vi "Check Step Result.vi"(7 "Execution in":refnum<data-value>, 8 "error in (no error)":errorcluster, 9 "Skipped":bool, 10 "Output Values in":cluster{"Name":string, "Variant Data":variant}[](array[cluster]), 11 "Step in":refnum<class "Step.lvclass">) -> (0 "Error Info":string, 1 "Result":T5, 2 "Measure Results":T2[](array[typedef]), 3 "Step out":refnum<class "Step.lvclass">, 4 "Value Limit Data":T1, 5 "Execution out":refnum<data-value>)   [LabVIEW 2015, in "Execution.lvclass"]
uses:
  Execution.lvclass
  Step.lvclass
  Step/STEP_STATUS.ctl
  STEP_MEASURE_RESULT.ctl
  Step/OUTPUT_DATA_TYPE.ctl
  OutputUI/OUTPUT_CHECK_TYPE.ctl
  <vilib>/Utility/error.llb/DialogType.ctl
panel:
  out "Output Values out":cluster{"Name":string, "Variant Data":variant}[](array[cluster])
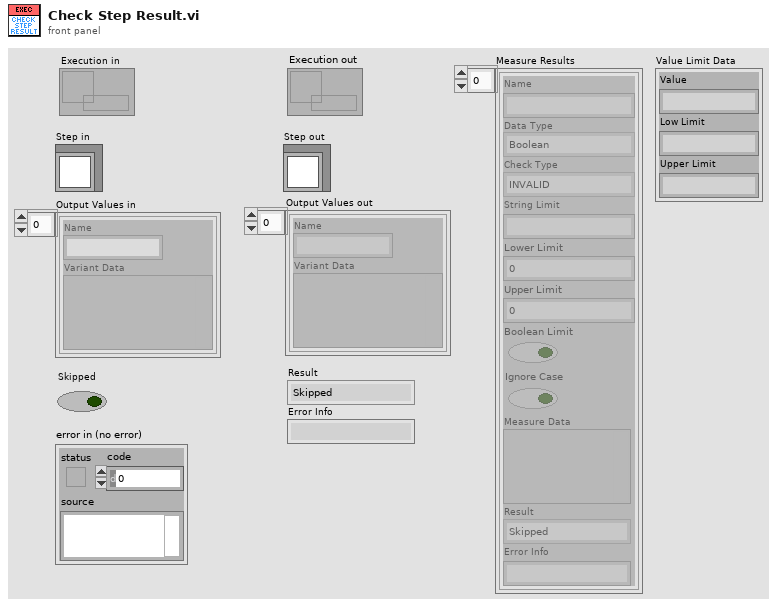
[diagram p1: front panel]
types:
  T1 = cluster{"Value":string, "Low Limit":string, "Upper Limit":string}
  T2 = typedef "Execution.lvclass/STEP_MEASURE_RESULT.ctl" = cluster{"Name":string, "Data Type":T3, "Check Type":T4, "String Limit":string, "Lower Limit":dbl, "Upper Limit":dbl, "Boolean Limit":bool, "Ignore Case":bool, "Measure Data":variant, "Result":T5, "Error Info":string}
  T3 = typedef "Step.lvclass/OUTPUT_DATA_TYPE.ctl" = enum16{"Boolean", "String", "Numeric", "Other"}
  T4 = typedef "Step.lvclass/OUTPUT_CHECK_TYPE.ctl" = enum16{"INVALID", "DO_NOT_CHECK", "RECORD", "VARIABLE", "EQUAL", "NOT_EQUAL", "STR_CONTAINS", "STR_START_WITH", "STR_END_WITH", "STR_REGEX_MATCH", "NUM_GT", "NUM_LT", "NUM_GE", "NUM_LE", "NUM_RANGE", "NUM_RANGE_BDY"}
  T5 = typedef "Step.lvclass/STEP_STATUS.ctl" = enum16{"Skipped", "Done", "Passed", "Failed", "Error"}
  T6 = typedef "Step.lvclass/STEP_OUTPUT.ctl" = cluster{"Label":string, "Name":string, "Data Type":T3, "Check Type":T4, "String Limit":string, "Lower Limit":dbl, "Upper Limit":dbl, "Boolean Limit":bool, "Ignore Case":bool, "Variable Name 1":string, "Limit Value Type 1":T7, "Variable Name 2":string, "Limit Value Type 2":T7}
  T7 = typedef "Step.lvclass/OUTPUT_VALUE_TYPE.ctl" = enum16{"Constant", "Variable"}
  T8 = typedef "DialogType.ctl" = u16
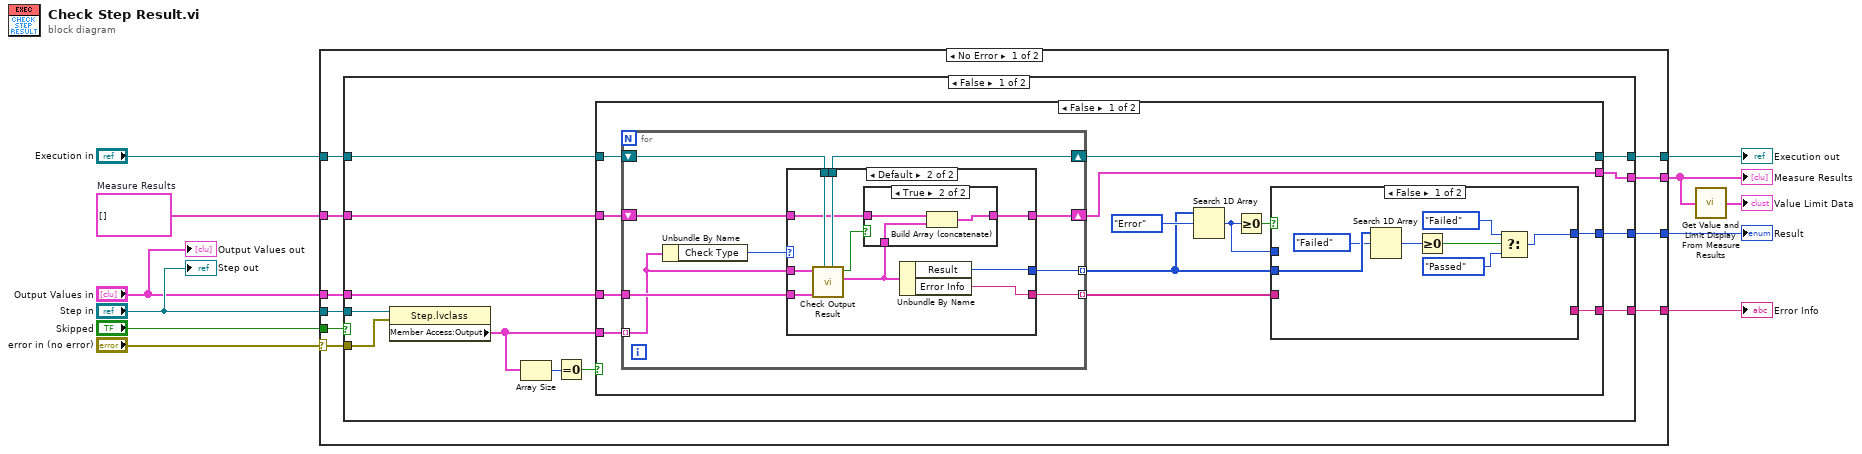
[diagram p0: block diagram]
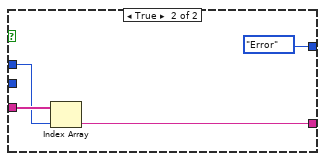
[diagram p2: hidden frame]
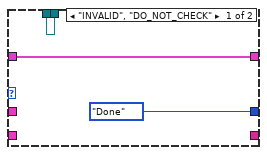
[diagram p3: hidden frame]
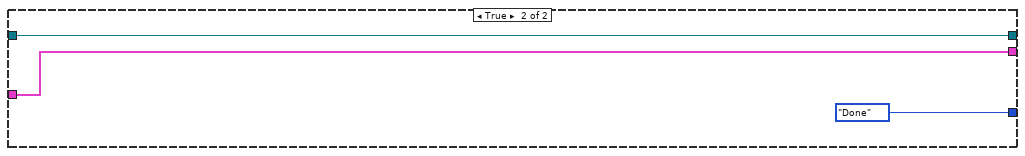
[diagram p5: hidden frame]
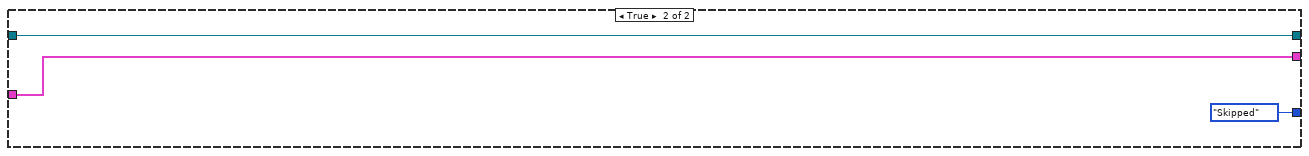
[diagram p6: hidden frame]
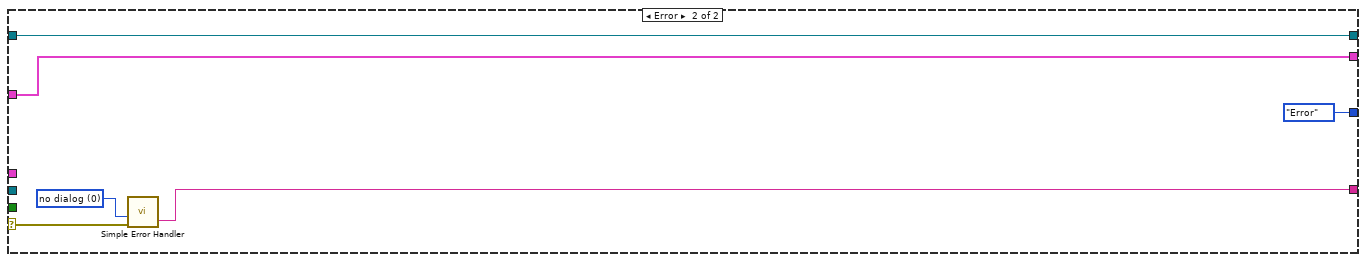
[diagram p7: hidden frame]
diagram:
  w3 = T2[] []  # Measure Results
  n1 = case shown="No Error" "error in (no error)" {
    selector: "error in (no error)" -> [w18 w94]
    tunnel: [w20 STEP_STATUS."Error" ("Status")] -> w10
    tunnel: [w16 w93] -> w9
    tunnel: "Skipped" -> [w21 _]
    tunnel: "Step in" -> [w19 _]
    tunnel: "Output Values in" -> [w17 _]
    tunnel: "Execution in" -> [w15 w91]
    tunnel: [w14 w91] -> w4
    tunnel: w3 -> [w13 w90]
    tunnel: [w12 w90] -> w2
    frame No Error {
      n2 = case shown="False" w21 {
        tunnel: [w29 STEP_STATUS."Skipped" ("Status")] -> w20
        tunnel: w19 -> [w33 _]
        tunnel: w18 -> [w32 _]
        tunnel: w17 -> [w27 _]
        tunnel: [w26 _] -> w16
        tunnel: w15 -> [w25 w88]
        tunnel: [w24 w88] -> w14
        tunnel: w13 -> [w23 w87]
        tunnel: [w22 w87] -> w12
        frame False {
          n3 = property class="Step.lvclass"(reference=w33, error in=w32) -> ("Member Access:Output"=w28:T6[])  [unwired: 2 out]
          n4 = Array Size(array=w28) -> (size(s)=w31:i32)
          n5 = Equal To 0?(x=w31) -> (x = 0?=w30:bool)
          n6 = case shown="False" w30 {
            tunnel: [w39 STEP_STATUS."Done" ("Status")] -> w29
            tunnel: w28 -> [w46 _]
            tunnel: w27 -> [w45 _]
            tunnel: [w38 _] -> w26
            tunnel: w25 -> [w37 w85]
            tunnel: [w36 w85] -> w24
            tunnel: w23 -> [w35 w84]
            tunnel: [w34 w84] -> w22
            frame False {
              n7 = for {
                tunnel: w46 -> [w61] mode=indexing
                tunnel: w45 -> [w66]
                tunnel: [w65] -> w40 mode=indexing
                tunnel: [w64] -> w41 mode=indexing
                shift-right: [w62] -> w36
                shift-left: w37 -> [w63]
                shift-right: [w58] -> w34
                shift-left: w35 -> [w59]
                n8 = Unbundle By Name(w61) -> ("Check Type"=w60:T4)
                n9 = case shown="Default" w60 {
                  tunnel: w61 -> [_ w79]
                  tunnel: w66 -> [_ w78]
                  tunnel: [STEP_STATUS."Done" ("Status") w72] -> w65
                  tunnel: [_ w71] -> w64
                  tunnel: w63 -> [w69 w77]
                  tunnel: [w69 w76] -> w62
                  tunnel: w59 -> [w67 w75]
                  tunnel: [w67 w74] -> w58
                  frame "INVALID", "DO_NOT_CHECK" {
                  }
                  frame Default {
                    n10 = call "Check Output Result.vi"("Execution in"=w77, "Output Values"=w78, "Step Output"=w79) -> ("Measure Result"=w73:T2, "Include In Result"=w70:bool, "Execution out"=w76:refnum<data-value>)  [unwired: 6 in]
                    n11 = case shown="True" w70 {
                      tunnel: w75 -> [w80 w83]
                      tunnel: [w80 w82] -> w74
                      tunnel: w73 -> [_ w81]
                      frame False {
                      }
                      frame True {
                        n12 = Build Array (concatenate)(w83, w81) -> (w82:T2[])
                      }
                    }
                    n13 = Unbundle By Name(w73) -> ("Result"=w72:T5, "Error Info"=w71:string)
                  }
                }
              }
              n14 = Search 1D Array(1D array=w40, element=STEP_STATUS."Error" ("Status")) -> (index of element=w42:i32)  [unwired: 1 in]
              n15 = Greater Or Equal To 0?(x=w42) -> (x >= 0?=w43:bool)
              n16 = case shown="False" w43 {
                tunnel: w42 -> [_ w56]
                tunnel: w41 -> [_ w57]
                tunnel: [w47 STEP_STATUS."Error" ("Status")] -> w39
                tunnel: [_ w54] -> w38
                tunnel: w40 -> [w53 _]
                frame False {
                  n17 = Search 1D Array(1D array=w53, element=STEP_STATUS."Failed" ("Status")) -> (index of element=w51:i32)  [unwired: 1 in]
                  n18 = Greater Or Equal To 0?(x=w51) -> (x >= 0?=w50:bool)
                  n19 = Select(t=STEP_STATUS."Failed" ("Status"), s=w50, f=STEP_STATUS."Passed" ("Status")) -> (s? t:f=w47:T5)
                }
                frame True {
                  n20 = Index Array(array=w57, index=w56) -> (element=w54:string)
                }
              }
            }
            frame True {
            }
          }
        }
        frame True {
        }
      }
    }
    frame Error {
      w92 = T8 0 items=["no dialog", "OK message", "continue or stop message", "OK message + warnings", "continue/stop + warnings"] ("type of dialog (OK msg:1)")
      n21 = call <vilib>:"Simple Error Handler.vi"("type of dialog (OK msg:1)"=w92, "error in (no error)"=w94) -> ("message"=w93:string)  [unwired: 3 in, 4 out]
    }
  }
  "Result" <- w10
  "Error Info" <- w9
  "Execution out" <- w4
  "Measure Results" <- w2
  n22 = call "Get Value and Limit Display From Measure Results.vi"("Measure Results"=w2) -> ("Value Limit Data"=→"Value Limit Data":T1)
  "Output Values out" <- "Output Values in"
  "Step out" <- "Step in"
